vi "WLAN - Test - UTIL - GenerateTestVectorFilePath.vi"(1 "Select Measurement":T1) -> (4 "TV Test Seq":path[](array[path]), 6 "TV Meas Config":path[](array[path]), 8 "TxSpectrumMeasurementsCSV":path[](array[path]), 10 "TxIQMeasurementsCSV":path[](array[path]))   [LabVIEW 2011]
uses:
  niWLAN/WLAN -  niWLAN - INC - Select Measurement.ctl
  <vilib>/Utility/file.llb/Write To Spreadsheet File (string).vi
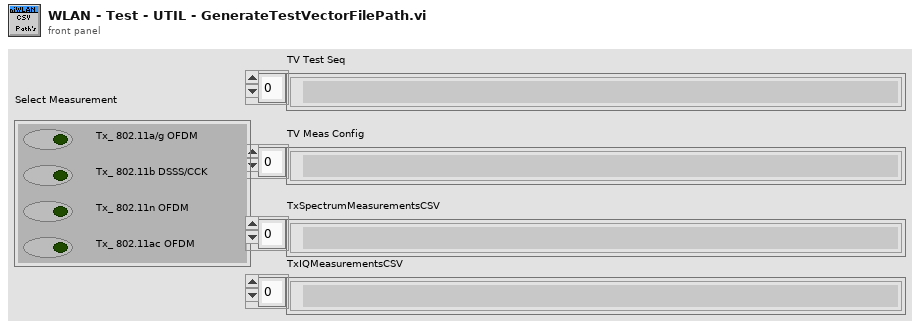
[diagram p1: front panel]
types:
  T1 = typedef "WLAN -  niWLAN - INC - Select Measurement.ctl" = cluster{"Tx_ 802.11a/g OFDM":bool, "Tx_ 802.11b DSSS/CCK":bool, "Tx_ 802.11n OFDM ":bool, "Tx_ 802.11ac OFDM ":bool}
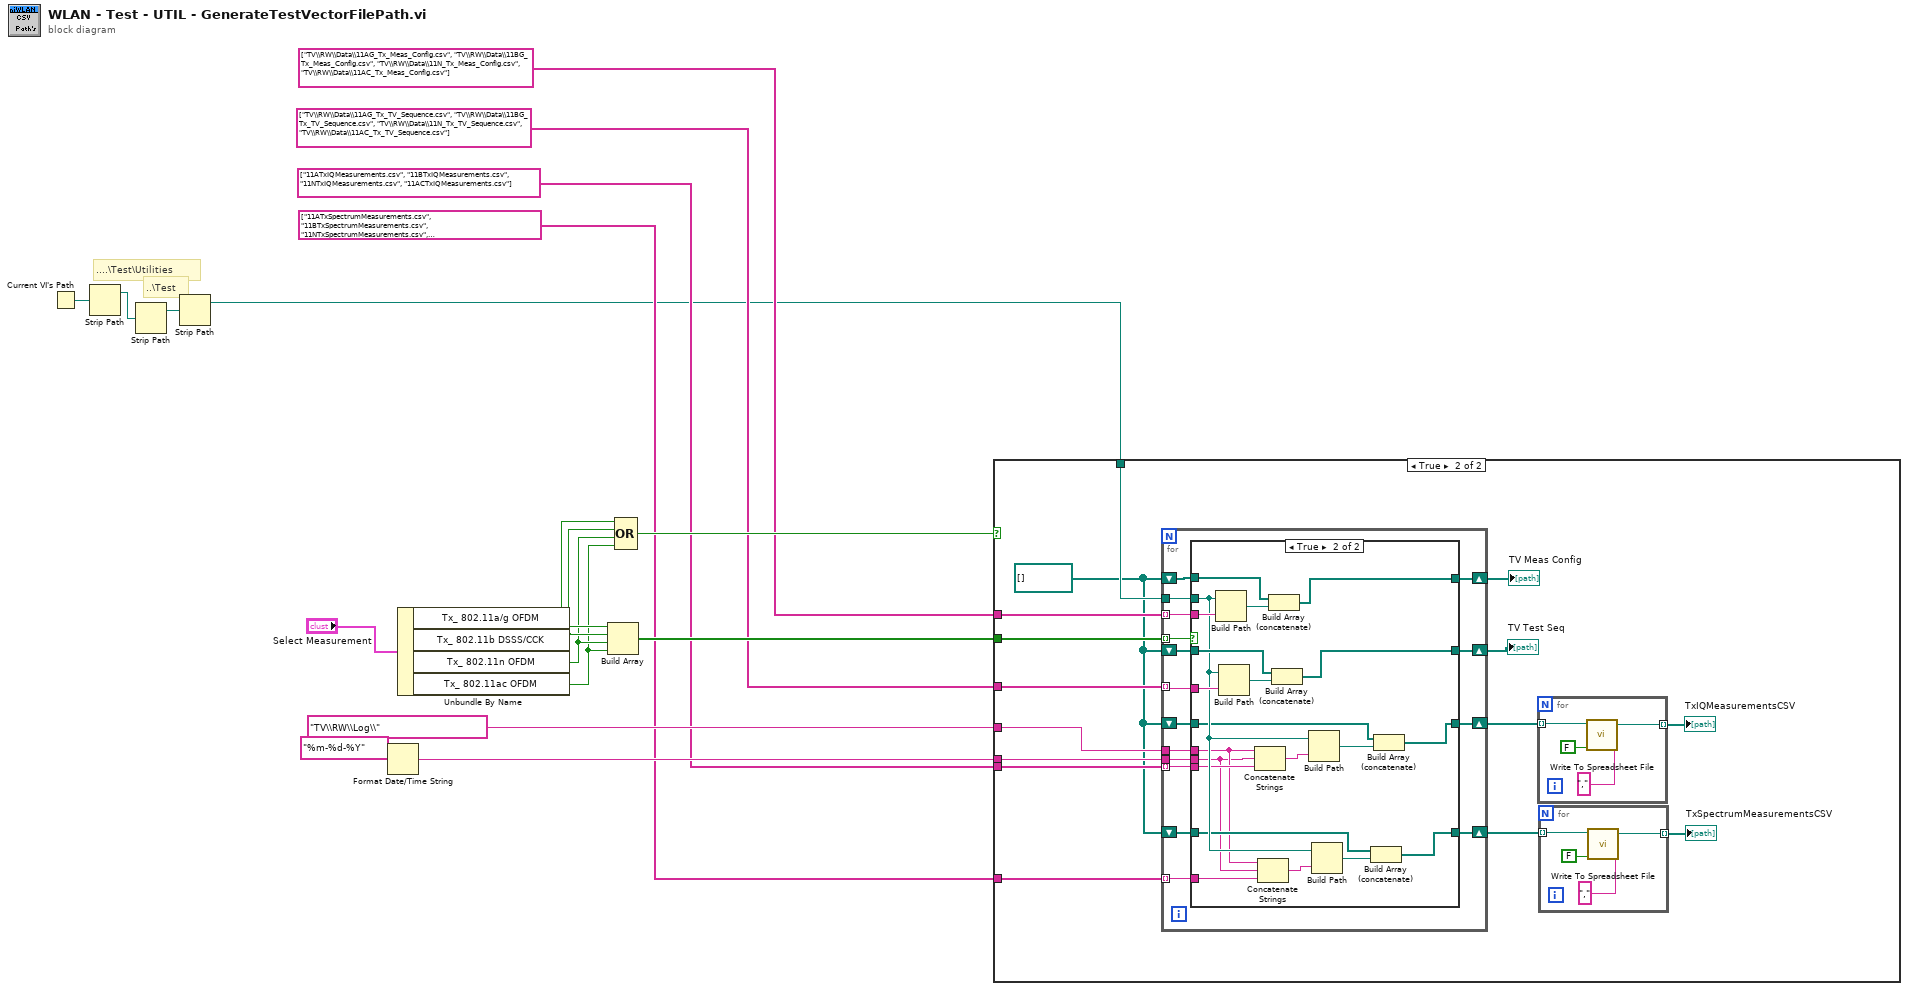
[diagram p0: block diagram]
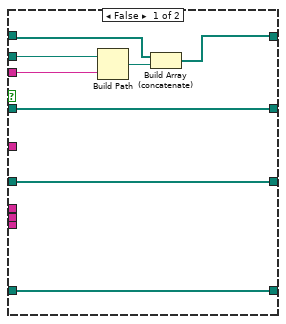
[diagram p3: hidden frame]
diagram:
  # "....\\Test\\Utilities"
  # "..\\Test"
  n1 = Current VI's Path() -> (path=w18:path)
  n2 = Strip Path(path=w18) -> (stripped path=w17:path)  [unwired: 1 out]
  n3 = Strip Path(path=w17) -> (stripped path=w16:path)  [unwired: 1 out]
  n4 = Strip Path(path=w16) -> (stripped path=w1:path)  [unwired: 1 out]
  n5 = Format Date/Time String(time format string (%c)="%m-%d-%Y") -> (date/time string=w13:string)  [unwired: 2 in]
  n6 = Unbundle By Name("Select Measurement") -> ("Tx_ 802.11a/g OFDM"=w9:bool, "Tx_ 802.11b DSSS/CCK"=w8:bool, "Tx_ 802.11n OFDM"=w7:bool, "Tx_ 802.11ac OFDM"=w6:bool)
  n7 = Build Array(w9, w8, w7, w6) -> (w5:bool[])
  n8 = Compound Arithmetic op=OR(w9, w8, w7, w6) -> (w11:bool)
  n9 = case shown="True" w11 {
    tunnel: "TV\\RW\\Log\\" ("name or relative path") -> [_ w23]
    tunnel: w13 -> [_ w22]
    tunnel: w1 -> [_ w21]
    tunnel: string[] ["TV\\RW\\Data\\11AG_Tx_Meas_Config.csv", "TV\\RW\\Data\\11BG_Tx_Meas_Config.csv", "TV\\RW\\Data\\11N_Tx_Meas_Config.csv", "TV\\RW\\Data\\11AC_Tx_Meas_Config.csv"] -> [_ w33]
    tunnel: w5 -> [_ w32]
    tunnel: string[] ["TV\\RW\\Data\\11AG_Tx_TV_Sequence.csv", "TV\\RW\\Data\\11BG_Tx_TV_Sequence.csv", "TV\\RW\\Data\\11N_Tx_TV_Sequence.csv", "TV\\RW\\Data\\11AC_Tx_TV_Sequence.csv"] -> [_ w30]
    tunnel: string[] ["11ATxSpectrumMeasurements.csv", "11BTxSpectrumMeasurements.csv", "11NTxSpectrumMeasurements.csv", "11ACTxSpectrumMeasurements.csv"] -> [_ w25]
    tunnel: string[] ["11ATxIQMeasurements.csv", "11BTxIQMeasurements.csv", "11NTxIQMeasurements.csv", "11ACTxIQMeasurements.csv"] -> [_ w24]
    frame False {
    }
    frame True {
      w20 = path[] []
      n10 = for {
        tunnel: w33 -> [w54] mode=indexing
        tunnel: w21 -> [w51]
        tunnel: w32 -> [w57] mode=indexing
        shift-right: [w56] -> w31
        shift-left: w20 -> [w55]
        shift-right: [w52] -> w19
        shift-left: w20 -> [w53]
        tunnel: w30 -> [w50] mode=indexing
        shift-right: [w49] -> w27
        shift-left: w20 -> [w48]
        shift-right: [w47] -> w26
        shift-left: w20 -> [w46]
        tunnel: w25 -> [w45] mode=indexing
        tunnel: w24 -> [w44] mode=indexing
        tunnel: w23 -> [w43]
        tunnel: w22 -> [w42]
        n11 = case shown="True" w57 {
          tunnel: w51 -> [w59 w76]
          tunnel: w54 -> [w58 w86]
          tunnel: [w61 w84] -> w56
          tunnel: w55 -> [w60 w83]
          tunnel: w53 -> [w65 w81]
          tunnel: [w65 w80] -> w52
          tunnel: w50 -> [_ w79]
          tunnel: [w63 w74] -> w49
          tunnel: w48 -> [w63 w73]
          tunnel: [w64 w71] -> w47
          tunnel: w46 -> [w64 w70]
          tunnel: w45 -> [_ w69]
          tunnel: w44 -> [_ w68]
          tunnel: w43 -> [_ w67]
          tunnel: w42 -> [_ w66]
          frame False {
            n12 = Build Path(base path=w59, name or relative path=w58) -> (appended path=w62:path)
            n13 = Build Array (concatenate)(w60, w62) -> (w61:path[])
          }
          frame True {
            n14 = Build Path(base path=w76, name or relative path=w86) -> (appended path=w85:path)
            n15 = Build Path(base path=w76, name or relative path=w79) -> (appended path=w82:path)
            n16 = Concatenate Strings(w67, w66, w68) -> (w78:string)
            n17 = Concatenate Strings(w67, w66, w69) -> (w77:string)
            n18 = Build Array (concatenate)(w83, w85) -> (w84:path[])
            n19 = Build Array (concatenate)(w81, w82) -> (w80:path[])
            n20 = Build Path(base path=w76, name or relative path=w78) -> (appended path=w75:path)
            n21 = Build Path(base path=w76, name or relative path=w77) -> (appended path=w72:path)
            n22 = Build Array (concatenate)(w70, w72) -> (w71:path[])
            n23 = Build Array (concatenate)(w73, w75) -> (w74:path[])
          }
        }
      }
      "TV Test Seq" <- w19
      "TV Meas Config" <- w31
      n24 = for {
        tunnel: [w41] -> w29 mode=indexing
        tunnel: w27 -> [w40] mode=indexing
        n25 = call-poly <vilib>:"Write To Spreadsheet File.vi"("delimiter (\\t)"="," ("delimiter (\\t)"), "append to file? (new file:F)"=FALSE, "file path (dialog if empty)"=w40) -> ("new file path (Not A Path if cancelled)"=w41:path)  [unwired: 5 in]
      }
      "TxIQMeasurementsCSV" <- w29
      n26 = for {
        tunnel: [w37] -> w28 mode=indexing
        tunnel: w26 -> [w36] mode=indexing
        n27 = call-poly <vilib>:"Write To Spreadsheet File.vi"("delimiter (\\t)"="," ("delimiter (\\t)"), "append to file? (new file:F)"=FALSE, "file path (dialog if empty)"=w36) -> ("new file path (Not A Path if cancelled)"=w37:path)  [unwired: 5 in]
      }
      "TxSpectrumMeasurementsCSV" <- w28
    }
  }
